vi "Write Input and Output Channel Count.vi"(8 "error in":errorcluster, 9 "number output channels":i32, 10 "number input channels":i32, 11 "digital input and output mode in":refnum<class "Digital Input and Output Mode.lvclass">) -> (0 "error out":errorcluster, 3 "digital input and output mode out":refnum<class "Digital Input and Output Mode.lvclass">)   [LabVIEW 2020, in "Scan Engine Scripting.lvlib" / "Digital Input and Output Mode.lvclass"]
uses:
  Digital Input and Output Mode.lvclass
  Digital Input and Output Mode.lvclass/Digital Input and Output Mode.ctl
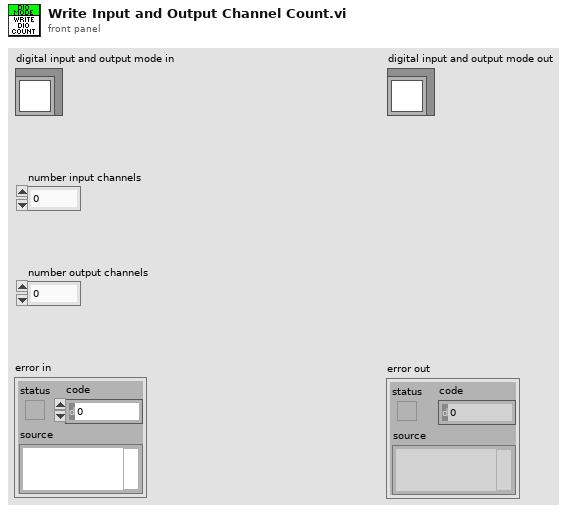
[diagram p1: front panel]
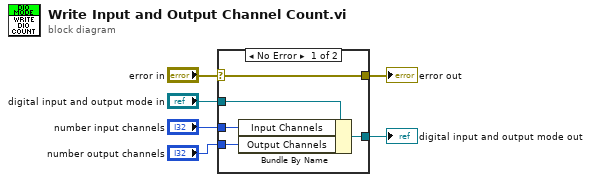
[diagram p0: block diagram]
diagram:
  n1 = case shown="No Error" "error in" {
    selector: "error in" -> [w10 w13]
    tunnel: [w10 w13] -> w5
    tunnel: [w9 w12] -> w3
    tunnel: "digital input and output mode in" -> [w11 w12]
    tunnel: "number output channels" -> [w8 _]
    tunnel: "number input channels" -> [w7 _]
    frame No Error {
      n2 = Bundle By Name(cluster=w11, "Input Channels"=w7, "Output Channels"=w8) -> (w9:refnum<class "Digital Input and Output Mode.lvclass">)
    }
    frame Error {
    }
  }
  "error out" <- w5
  "digital input and output mode out" <- w3
